vi "Read Events.vi"(8 "error in (no error)":errorcluster, 11 "Event_Source in":refnum<class "Event_Source.lvclass">) -> (0 "error out":errorcluster, 2 "Events":refnum<class "Event_Polled Type.lvclass">[](array[class]), 3 "Event_Source out":refnum<class "Event_Source.lvclass">)   [LabVIEW 2021, in "Event_Source.lvclass"]
uses:
  Event_Source.lvclass
  Event_Source.lvclass/Event_Source.ctl
  Event_Polled Type.lvclass
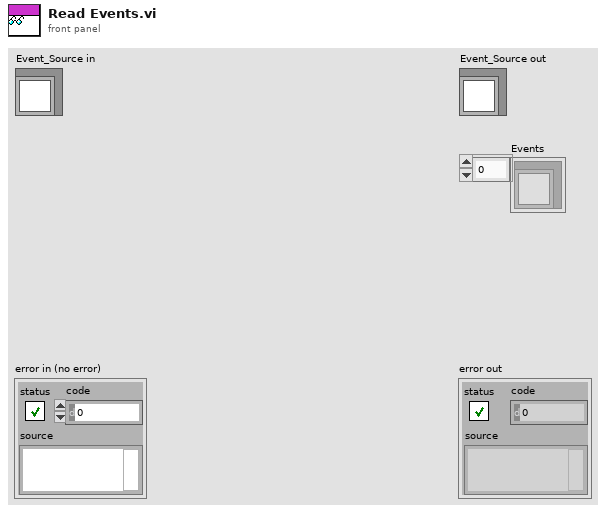
[diagram p1: front panel]
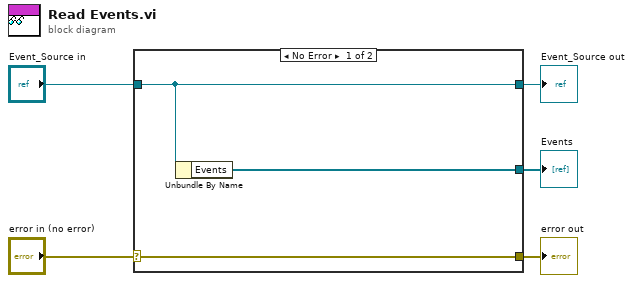
[diagram p0: block diagram]
diagram:
  n1 = case shown="No Error" "error in (no error)" {
    selector: "error in (no error)" -> [w8 w9]
    tunnel: [w8 w9] -> w4
    tunnel: [w7 w10] -> w2
    tunnel: "Event_Source in" -> [w7 w10]
    tunnel: [w6 _] -> w1
    frame No Error {
      n2 = Unbundle By Name(w7) -> ("Events"=w6:refnum<class "Event_Polled Type.lvclass">[])
    }
    frame Error {
    }
  }
  "error out" <- w4
  "Event_Source out" <- w2
  "Events" <- w1
